vi "Add Response.vi"   [LabVIEW 2018, in "Instrument Addon Scripting API.lvlib"]
uses:
  Instrument Addon Scripting API.lvlib
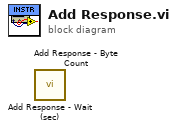
[diagram p0: block diagram]
diagram:
  n1 = call "Add Response - Wait (sec).vi"() -> ()  [unwired: 12 in]
  n2 = call "Add Response - Byte Count.vi"() -> ()  [unwired: 12 in]
